vi "String To Array Test.vi"(11 "Error In":errorcluster) -> (15 "Error Out":errorcluster)   [LabVIEW 2021, in "Test Files.lvlib"]
doc: "This VI has test cases for checking the functionality of String To Array.vi"
uses:
  Test Files.lvlib
  CustomSortPath.lvlib
  <vilib>/addons/_JKI Toolkits/Caraya/classes/Test/Test.lvclass
  <vilib>/addons/_JKI Toolkits/Caraya/classes/Assert/Assert.lvclass
  <vilib>/addons/_JKI Toolkits/Caraya/classes/Assert/Assert Equal Value_Variant.vi
panel:
  # "String to array test"
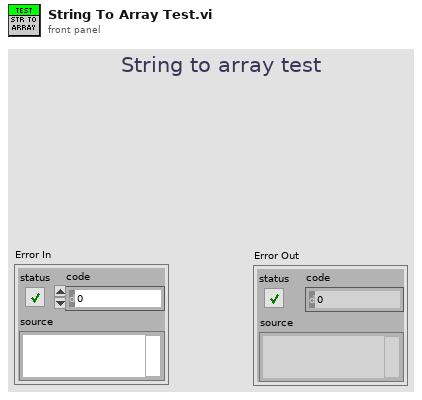
[diagram p1: front panel]
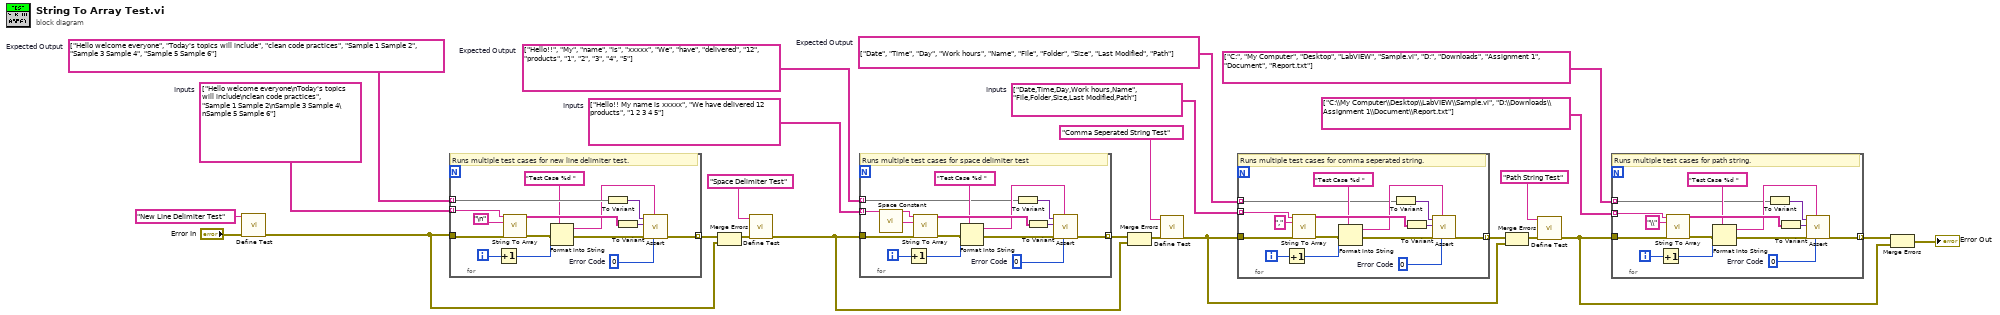
[diagram p0: block diagram]
diagram:
  w16 = string[][] [["Date", "Time", "Day", "Work hours", "Name"], ["File", "Folder", "Size", "Last Modified", "Path"]]  # Expected Output
  w20 = string[][] [["Hello!!", "My", "name", "is", "xxxxx"], ["We", "have", "delivered", "12", "products"], ["1", "2", "3", "4", "5"]]  # Expected Output
  w22 = string[][] [["Hello welcome everyone", "Today's topics will include", "clean code practices"], ["Sample 1 Sample 2", "Sample 3 Sample 4", "Sample 5 Sample 6"]]  # Expected Output
  w17 = string[] ["Date,Time,Day,Work hours,Name", "File,Folder,Size,Last Modified,Path"]  # Inputs
  w19 = string[] ["Hello!! My name is xxxxx", "We have delivered 12 products", "1 2 3 4 5"]  # Inputs
  w23 = string[] ["Hello welcome everyone\nToday's topics will include\nclean code practices", "Sample 1 Sample 2\nSample 3 Sample 4\nSample 5 Sample 6"]  # Inputs
  n1 = call <vilib>:"Define Test.vi"("error in (no error)"="Error In", "Label (VI Title)"="New Line Delimiter Test") -> ("error out"=w10:errorcluster)  [unwired: 8 in, 1 out]
  n2 = for {
    tunnel: w23 -> [w38] mode=indexing
    tunnel: w22 -> [w35] mode=indexing
    tunnel: w10 -> [w40]
    tunnel: [w27] -> w11 mode=indexing
    i -> [w33]
    w26 = 0  # Error Code
    # "Runs multiple test cases for new line delimiter test."
    n3 = Increment(x=w33) -> (x+1=w31:i32)
    n4 = call "String To Array.vi"("String"=w38, "delimiter (Tab)"="\n", "error in (no error)"=w40) -> ("1DArray"=w37:string[], "error out"=w32:errorcluster)  [unwired: 11 in]
    n5 = Format Into String(format string="Test Case %d ", error in=w32, w31) -> (resulting string=w29:string, error out=w28:errorcluster)  [unwired: 1 in]
    n6 = To Variant(anything=w35) -> (Variant=w34:variant)
    n7 = To Variant(anything=w37) -> (Variant=w36:variant)
    n8 = call-poly <vilib>:"Assert.vi"("error code (1)"=w26, "Label"=w29, "error in (no error)"=w28, "Y"=w36, "X"=w34) -> ("error out"=w27:errorcluster)  [unwired: 5 in, 1 out]
  }
  n9 = Merge Errors(w11, w10) -> (w12:errorcluster)
  n10 = call <vilib>:"Define Test.vi"("error in (no error)"=w12, "Label (VI Title)"="Space Delimiter Test") -> ("error out"=w7:errorcluster)  [unwired: 8 in, 1 out]
  n11 = for {
    tunnel: w20 -> [w44] mode=indexing
    tunnel: w19 -> [w43] mode=indexing
    tunnel: w7 -> [w55]
    tunnel: [w45] -> w8 mode=indexing
    i -> [w51]
    w41 = 0  # Error Code
    # "Runs multiple test cases for space delimiter test"
    n12 = call <vilib>:"Space Constant.vi"() -> ("String"=w42:string)
    n13 = Increment(x=w51) -> (x+1=w49:i32)
    n14 = call "String To Array.vi"("String"=w43, "delimiter (Tab)"=w42, "error in (no error)"=w55) -> ("1DArray"=w54:string[], "error out"=w50:errorcluster)  [unwired: 11 in]
    n15 = Format Into String(format string="Test Case %d ", error in=w50, w49) -> (resulting string=w47:string, error out=w46:errorcluster)  [unwired: 1 in]
    n16 = To Variant(anything=w44) -> (Variant=w52:variant)
    n17 = To Variant(anything=w54) -> (Variant=w53:variant)
    n18 = call-poly <vilib>:"Assert.vi"("error code (1)"=w41, "Label"=w47, "error in (no error)"=w46, "Y"=w53, "X"=w52) -> ("error out"=w45:errorcluster)  [unwired: 5 in, 1 out]
  }
  n19 = Merge Errors(w8, w7) -> (w9:errorcluster)
  n20 = call <vilib>:"Define Test.vi"("error in (no error)"=w9, "Label (VI Title)"="Comma Seperated String Test") -> ("error out"=w4:errorcluster)  [unwired: 8 in, 1 out]
  n21 = for {
    tunnel: w17 -> [w59] mode=indexing
    tunnel: w16 -> [w57] mode=indexing
    tunnel: w4 -> [w70]
    tunnel: [w60] -> w5 mode=indexing
    i -> [w66]
    w56 = 0  # Error Code
    # "Runs multiple test cases for comma seperated string."
    n22 = Increment(x=w66) -> (x+1=w64:i32)
    n23 = call "String To Array.vi"("String"=w59, "delimiter (Tab)"=",", "error in (no error)"=w70) -> ("1DArray"=w69:string[], "error out"=w65:errorcluster)  [unwired: 11 in]
    n24 = Format Into String(format string="Test Case %d ", error in=w65, w64) -> (resulting string=w62:string, error out=w61:errorcluster)  [unwired: 1 in]
    n25 = To Variant(anything=w57) -> (Variant=w67:variant)
    n26 = To Variant(anything=w69) -> (Variant=w68:variant)
    n27 = call-poly <vilib>:"Assert.vi"("error code (1)"=w56, "Label"=w62, "error in (no error)"=w61, "Y"=w68, "X"=w67) -> ("error out"=w60:errorcluster)  [unwired: 5 in, 1 out]
  }
  n28 = Merge Errors(w5, w4) -> (w6:errorcluster)
  n29 = call <vilib>:"Define Test.vi"("error in (no error)"=w6, "Label (VI Title)"="Path String Test") -> ("error out"=w1:errorcluster)  [unwired: 8 in, 1 out]
  n30 = for {
    tunnel: string[] ["C:\\My Computer\\Desktop\\LabVIEW\\Sample.vi", "D:\\Downloads\\Assignment 1\\Document\\Report.txt"] -> [w72] mode=indexing
    tunnel: string[][] [["C:", "My Computer", "Desktop", "LabVIEW", "Sample.vi"], ["D:", "Downloads", "Assignment 1", "Document", "Report.txt"]] ("appended array") -> [w73] mode=indexing
    tunnel: w1 -> [w85]
    tunnel: [w75] -> w3 mode=indexing
    i -> [w81]
    w71 = 0  # Error Code
    # "Runs multiple test cases for path string."
    n31 = Increment(x=w81) -> (x+1=w79:i32)
    n32 = call "String To Array.vi"("String"=w72, "delimiter (Tab)"="\\", "error in (no error)"=w85) -> ("1DArray"=w84:string[], "error out"=w80:errorcluster)  [unwired: 11 in]
    n33 = Format Into String(format string="Test Case %d ", error in=w80, w79) -> (resulting string=w77:string, error out=w76:errorcluster)  [unwired: 1 in]
    n34 = To Variant(anything=w73) -> (Variant=w82:variant)
    n35 = To Variant(anything=w84) -> (Variant=w83:variant)
    n36 = call-poly <vilib>:"Assert.vi"("error code (1)"=w71, "Label"=w77, "error in (no error)"=w76, "Y"=w83, "X"=w82) -> ("error out"=w75:errorcluster)  [unwired: 5 in, 1 out]
  }
  n37 = Merge Errors(w3, w1) -> (→"Error Out":errorcluster)
